vi "Method 3.vi"(10 "My Input":dbl, 11 "Test Interface in":refnum<class "Test Interface.lvclass">) -> (2 "My Output":dbl, 3 "Test Interface out":refnum<class "Test Interface.lvclass">)   [LabVIEW 2023, in "Test Interface.lvlib" / "Test Interface.lvclass"]
doc: "My Method Description"
uses:
  Test Interface.lvclass
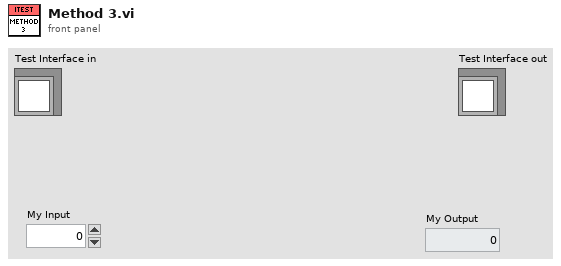
[diagram p1: front panel]
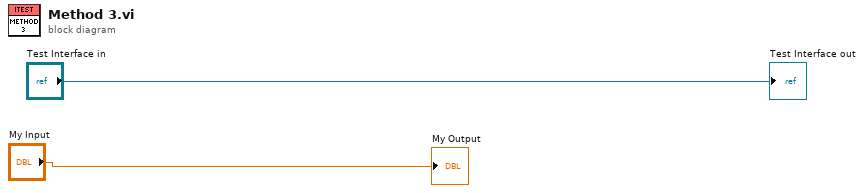
[diagram p0: block diagram]
diagram:
  "Test Interface out" <- "Test Interface in"
  "My Output" <- "My Input"
